vi "Dispose Image Spaces.vi"(8 "error in (no error)":errorcluster, 11 "[Images]":T1[](array[typedef])) -> (0 "error out":errorcluster)   [LabVIEW 2013]
doc: "Disposes the image spaces."
uses:
  <vilib>/vision/Image Controls.llb/IMAQ Image.ctl
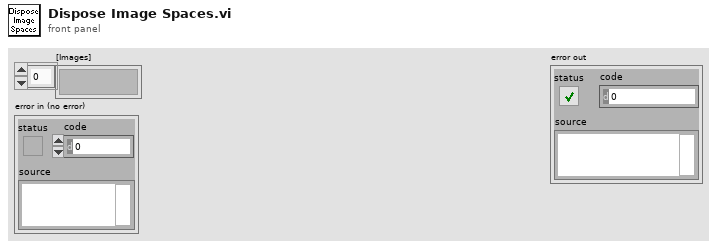
[diagram p1: front panel]
types:
  T1 = typedef "IMAQ Image.ctl" = refnum<image>
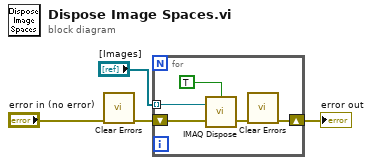
[diagram p0: block diagram]
diagram:
  n1 = call <vilib>:"Clear Errors.vi"("error in (no error)"="error in (no error)") -> ("error out"=w4:errorcluster)  [unwired: 6 in]
  n2 = for {
    tunnel: "[Images]" -> [w9] mode=indexing
    shift-right: [w5] -> w1
    shift-left: w4 -> [w7]
    n3 = call "IMAQ Dispose"("All Images? (No)"=TRUE, "Image"=w9, "error in (no error)"=w7) -> ("error out"=w6:errorcluster)  [unwired: 3 in]
    n4 = call <vilib>:"Clear Errors.vi"("error in (no error)"=w6) -> ("error out"=w5:errorcluster)  [unwired: 6 in]
  }
  "error out" <- w1
